vi "char2bit.vi"(10 "输入要传输的信息":string="hello,my name is liuxiaowei") -> (1 "用户信息大小":i32, 2 "输出比特信息":i8[](array[numeric]))   [LabVIEW 2010]
panel:
  out "大小":i32[](array[numeric])
  out "值":u8[](array[numeric])
  out "数据字符串":string
  out "数组":i8[](array[numeric])
  out "数值":i32
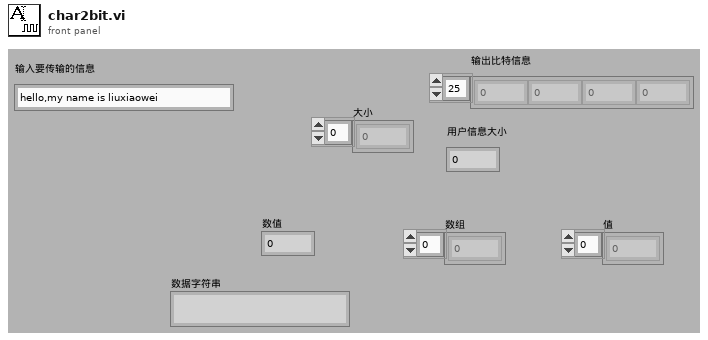
[diagram p1: front panel]
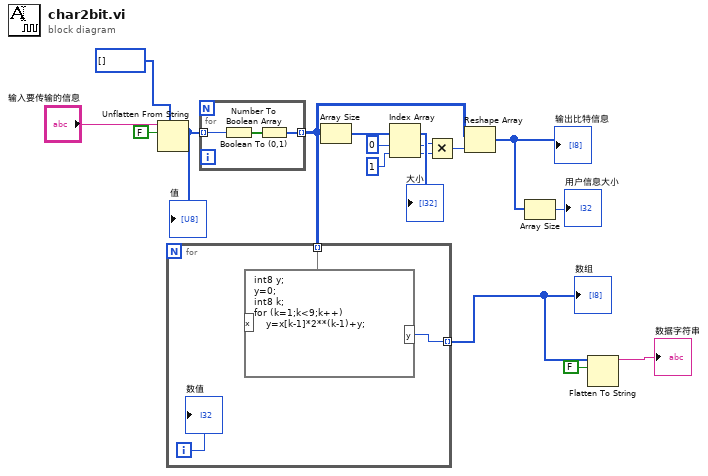
[diagram p0: block diagram]
diagram:
  n1 = Unflatten From String(type=u8[] [], binary string="输入要传输的信息", data includes array or string size? (T)=FALSE ("数据中包含数组或字符串大小？(T)")) -> (value=w5:u8[])  [unwired: 2 in, 2 out]
  "值" <- w5
  n2 = for {
    tunnel: w5 -> [w19] mode=indexing
    tunnel: [w17] -> w1 mode=indexing
    n3 = Number To Boolean Array(number=w19) -> (Boolean array=w18:bool[])
    n4 = Boolean To (0,1)(Boolean=w18) -> (0, 1=w17:i16[])
  }
  n5 = for {
    tunnel: [w21] -> w4 mode=indexing
    tunnel: w1 -> [w20] mode=indexing
    i -> [w22]
    n6 = formula code="int8 y;\ny=0;\nint8 k;\nfor (k=1;k<9;k++)\n    y=x[k-1]*2**(k-1)+y;"("x"=w20) -> ("y"=w21:i8)
    "数值" <- w22
  }
  "数组" <- w4
  n7 = Array Size(array=w1) -> (size(s)=w14:i32[])
  "大小" <- w14
  n8 = Index Array(array=w14, index #1=0 ("索引"), index #2=1 ("索引")) -> (element #1=w11:i32, element #2=w10:i32)
  n9 = Multiply(x=w11, y=w10) -> (x*y=w9:i32)
  n10 = Reshape Array(w1, w9) -> (w7:i16[])
  "输出比特信息" <- w7
  n11 = Array Size(array=w7) -> (size(s)=→"用户信息大小":i32)
  n12 = Flatten To String(anything=w4, prepend array or string size? (T)=FALSE ("预置数组或字符串大小？(T)")) -> (data string=→"数据字符串":string)  [unwired: 2 in, 2 out]
